vi "Der_Linear.vi"(1 "g'(z)":T1, 2 "dA_l":T1) -> (0 "dZ_l":T1)   [LabVIEW 2016]
uses:
  <vilib>/Analysis/Matrix/Datatypes/RealMatrix.ctl
  <vilib>/Analysis/Matrix/Numeric/Conversions/Matrix To Array - RM.vi
  <vilib>/Analysis/Matrix/Numeric/Conversions/Array To Matrix - RA2.vi
  <vilib>/Analysis/Matrix/NI_Matrix.lvlib
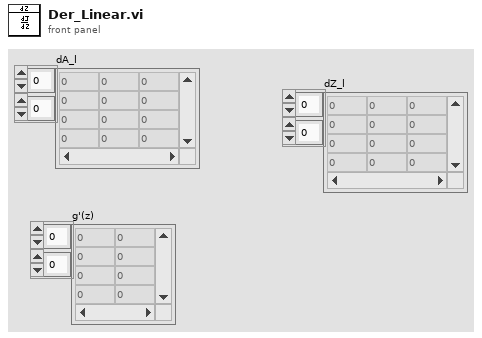
[diagram p1: front panel]
types:
  T1 = typedef "NI_Matrix.lvlib/RealMatrix.ctl" = dbl[][]
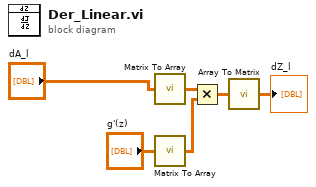
[diagram p0: block diagram]
diagram:
  n1 = call-poly <vilib>:"Matrix To Array.vi"("Real Matrix"="dA_l") -> ("Real 2D Array"=w5:dbl[][])
  n2 = call-poly <vilib>:"Matrix To Array.vi"("Real Matrix"="g'(z)") -> ("Real 2D Array"=w4:dbl[][])
  n3 = Multiply(x=w5, y=w4) -> (x*y=w3:dbl[][])
  n4 = call-poly <vilib>:"Array To Matrix.vi"("Real 2D Array"=w3) -> ("Real Matrix"=→"dZ_l":T1)
